vi "直通基准测试.vi"(8 "error in (no error)":errorcluster, 9 "out":i32=1, 11 "in":i32=2) -> (0 "error out":errorcluster)   [LabVIEW 2015]
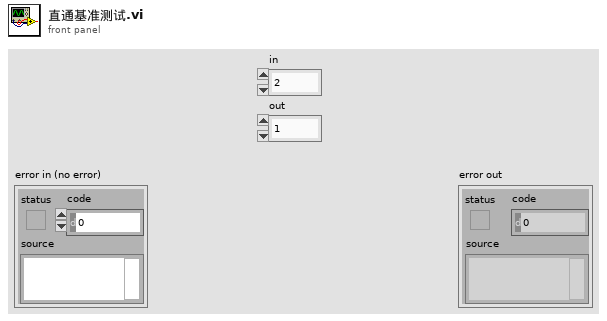
[diagram p1: front panel]
types:
  T1 = typedef "直通基准state.ctl" = enum16{"Idle", "开始消息", "切换开关", "网分测量", "数据库操作", "结束消息"}
  T2 = cluster{"Freq":dbl[], "S11":dbl[], "S12":dbl[], "S21":dbl[], "S22":dbl[]}
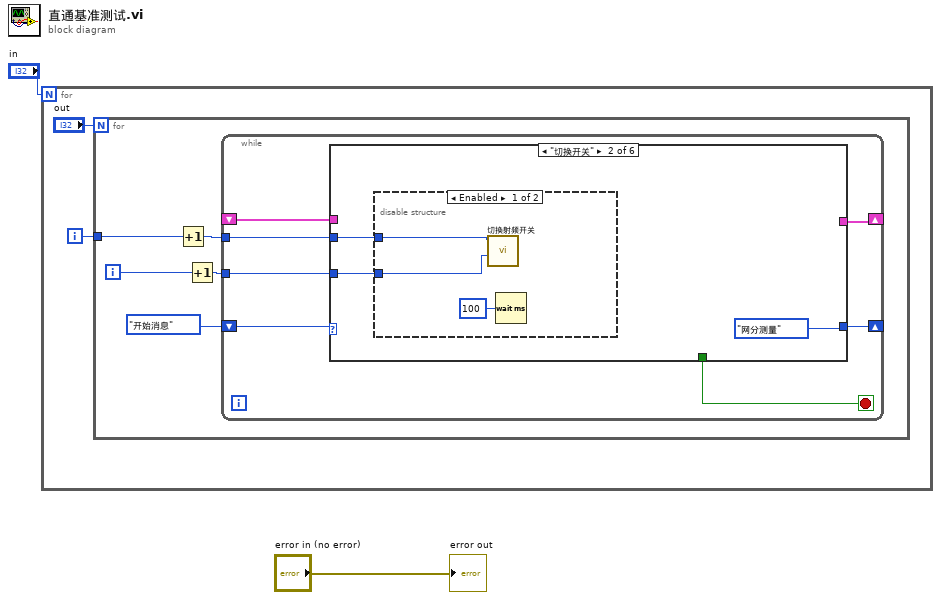
[diagram p0: block diagram]
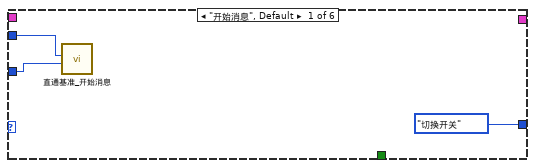
[diagram p2: hidden frame]
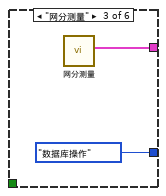
[diagram p4: hidden frame]
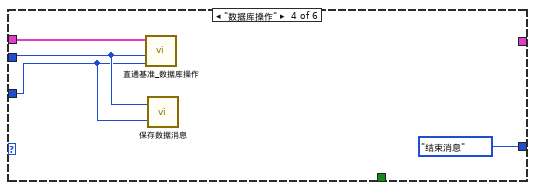
[diagram p5: hidden frame]
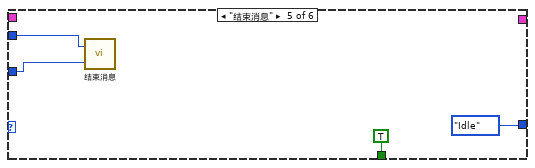
[diagram p6: hidden frame]
diagram:
  n1 = for {
    N: "in" -> [_]
    i -> [w3]
    n2 = for {
      N: "out" -> [_]
      tunnel: w3 -> [w9]
      i -> [w8]
      n3 = Increment(x=w9) -> (x+1=w7:i32)
      n4 = Increment(x=w8) -> (x+1=w6:i32)
      n5 = while {
        tunnel: w7 -> [w16]
        tunnel: w6 -> [w15]
        shift-right: [w13] -> _
        shift-left: 直通基准state."开始消息" ("直通基准State") -> [w14]
        shift-right: [w11] -> _
        shift-left: _ -> [w10]
        stop <- w12 stop-if-true
        n6 = case shown="\"切换开关\"" w14 {
          tunnel: w16 -> [w18 w22 _ w29 w33 _]
          tunnel: w15 -> [w17 w21 _ w28 w32 _]
          tunnel: [直通基准state."切换开关" ("直通基准State") 直通基准state."网分测量" ("直通基准State") 直通基准state."数据库操作" ("直通基准State") 直通基准state."结束消息" ("直通基准State") 直通基准state."Idle" ("直通基准State") _] -> w13
          tunnel: [_ _ _ _ TRUE _] -> w12
          tunnel: [_ _ w27 _ _ _] -> w11
          tunnel: w10 -> [_ _ _ w31 _ _]
          frame "开始消息", Default {
            n7 = call "直通基准_开始消息.vi"("COM"=w17, "A"=w18) -> ()  [unwired: 10 in]
          }
          frame "切换开关" {
            n8 = disable-structure shown="Enabled" {
              disable-tunnel: w22 -> [w24 _]
              disable-tunnel: w21 -> [w23 _]
              frame Enabled {
                n9 = call "切换射频开关.vi"("COM"=w23, "A"=w24) -> ()  [unwired: 7 in, 3 out]
                n10 = Wait (ms)(milliseconds to wait=u32 100) -> ()  [unwired: 1 out]
              }
              frame Disabled {
              }
            }
          }
          frame "网分测量" {
            n11 = call "网分测量.vi"() -> ("Freq&S"=w27:T2)  [unwired: 11 in]
          }
          frame "数据库操作" {
            n12 = call "直通基准_数据库操作.vi"("出口"=w28, "进口"=w29, "Freq&S"=w31) -> ()  [unwired: 9 in]
            n13 = call "保存数据消息.vi"("COM"=w28, "A"=w29) -> ()  [unwired: 1 in]
          }
          frame "结束消息" {
            n14 = call "结束消息.vi"("COM"=w32, "A"=w33) -> ()  [unwired: 1 in]
          }
          frame "Idle" {
          }
        }
      }
    }
  }
  "error out" <- "error in (no error)"
